vi "Calibratge.vi"() -> (1 "OK ?":bool)   [LabVIEW 2017]
uses:
  <vilib>/registry/registry.llb/Registry RtKey.ctl
  <vilib>/registry/registry.llb/Registry View.ctl
  <vilib>/registry/registry.llb/Write Registry Value Simple STR.vi
panel:
  in  "TermeInd 2":dbl caption="PendentCel2"
  out "TermesInd":dbl[](array[numeric]) caption="Pendents" format="%#_8g"
  in  "TermeInd 1":dbl caption="PendentCel1"
  in  "CALIBRAR":bool caption="ACTIVA CALIBRAR"
  in  "Idioma":string(combo)
  in  "ViuMotor":bool caption="Viu Motor Actiu"
  in  "MotorBipolar":bool caption="Motor Bipolar"
  in  "DeforActiva":bool
  in  "VelocitatMaxima":dbl caption="Velocitat Màxima"
  in  "ResoExten":i8(ring) caption="Resolució Extensometre" items=["0.1", "0.2", "0.5", "0.01", "0.02", "0.05", "0.001", "0.002", "0.005"]
  in  "Pendent_D":dbl caption="Extensometro" format="%#_8g"
  in  "Text Defor":string caption="Text defor"
  out "Unidades 2":i32[](array[numeric])
  in  "Unidades Célula 2":i32[](listbox) caption="Célula 2"
  out "Unidades 1":i32[](array[numeric])
  in  "Célula 2":u8(ring) items=["0.5 kg", "1 Kg", "2 Kg", "5 kg", "10 kg", "20 kg", "50 kg", "100 kg", "200 kg", "300 kg", "500 kg", "1000 kg", "2000 kg", "5000 kg", "10000 kg", "20000 kg", "30000 kg", "P-20 kg", "P-200 kg", "P-500 kg", "P-5000 kg", "P-20000 kg", "P-40 bar", "P-60 bar", "P- 20 bar", "No presente"]
  in  "Unidades Célula 1":i32[](listbox) caption="Célula 1"
  in  "SobrecargaC2":dbl
  in  "SobrecargaC1":dbl
  in  "C3-E2":u16(ring) items=["1", "2", "5", "10", "0.1", "0.01", "0.001", "0.0001", "0.5", "0.05", "0.005", "0.0005", "0.25", "0.025", "0.0025", "0.00025", "0.2", "0.02", "0.002", "0.0002"]
  in  "C2-E2":u16(ring) items=["1", "2", "5", "10", "0.1", "0.01", "0.001", "0.0001", "0.5", "0.05", "0.005", "0.0005", "0.25", "0.025", "0.0025", "0.00025", "0.2", "0.02", "0.002", "0.0002"]
  in  "C3-E1":u16(ring) items=["1", "2", "5", "10", "0.1", "0.01", "0.001", "0.0001", "0.5", "0.05", "0.005", "0.0005", "0.25", "0.025", "0.0025", "0.00025", "0.2", "0.02", "0.002", "0.0002"]
  in  "C2-E1":u16(ring) items=["1", "2", "5", "10", "0.1", "0.01", "0.001", "0.0001", "0.5", "0.05", "0.005", "0.0005", "0.25", "0.025", "0.0025", "0.00025", "0.2", "0.02", "0.002", "0.0002"]
  out "Célula 3":string
  in  "PendentCel3":dbl
  in  "PendentCel2":dbl
  in  "Número de Célules":dbl
  in  "TextTemps":string caption="Text temps"
  in  "Célula 1":i8(ring) items=["0.5 kg", "1 Kg", "2 Kg", "5 kg", "10 kg", "20 kg", "50 kg", "100 kg", "200 kg", "300 kg", "500 kg", "1000 kg", "2000 kg", "5000 kg", "10000 kg", "20000 kg", "30000 kg", "P-20 kg", "P-200 kg", "P-500 kg", "P-5000 kg", "P-20000 kg", "P-40 bar", "P-60 bar", "P-20 bar"]
  in  "PendentCel1":dbl
  in  "Password":string
  in  "error in (no error)":errorcluster
  out "Pendents":dbl[](array[numeric]) format="%#_8g"
  in  "Cancel":bool
  in  "OK Button":bool
  in  "Pendent_T":dbl caption="CaptadorD" format="%#_8g"
  # "Pendent"
  # "Sobrecarga"
  # "Ind."
  # "Pendent"
  # "Sobrecarga"
  # "Si vols modificar el password\nintrodueix-ne un de nou"
  # "Ind."
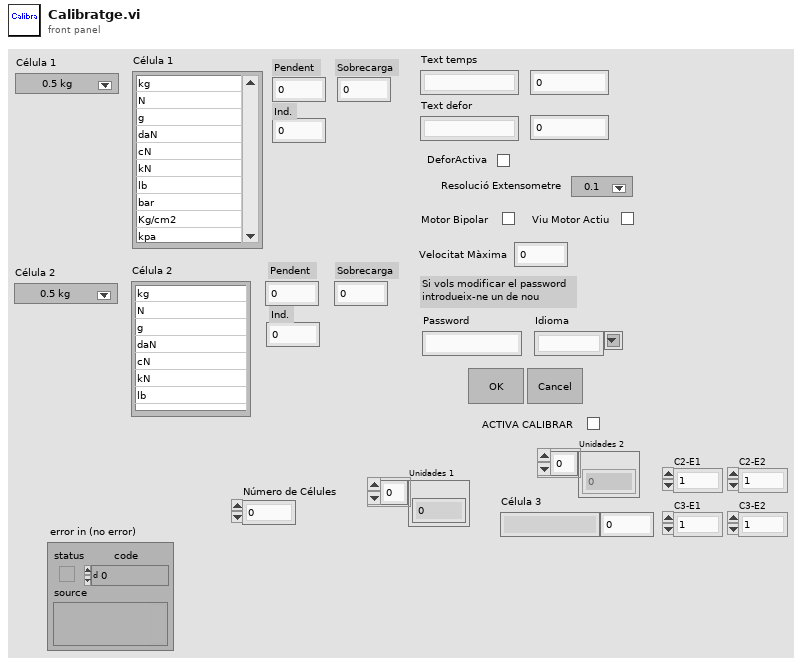
[diagram p1: front panel]
types:
  T1 = typedef "Registry RtKey.ctl" = enum32{"HKEY_CLASSES_ROOT", "HKEY_CURRENT_USER", "HKEY_LOCAL_MACHINE", "HKEY_USERS", "HKEY_PERFORMANCE_DATA", "HKEY_CURRENT_CONFIG", "HKEY_DYN_DATA"}
  T2 = typedef "Registry View.ctl" = u16
  T3 = typedef "Registry refnum.ctl" = refnum<k1>
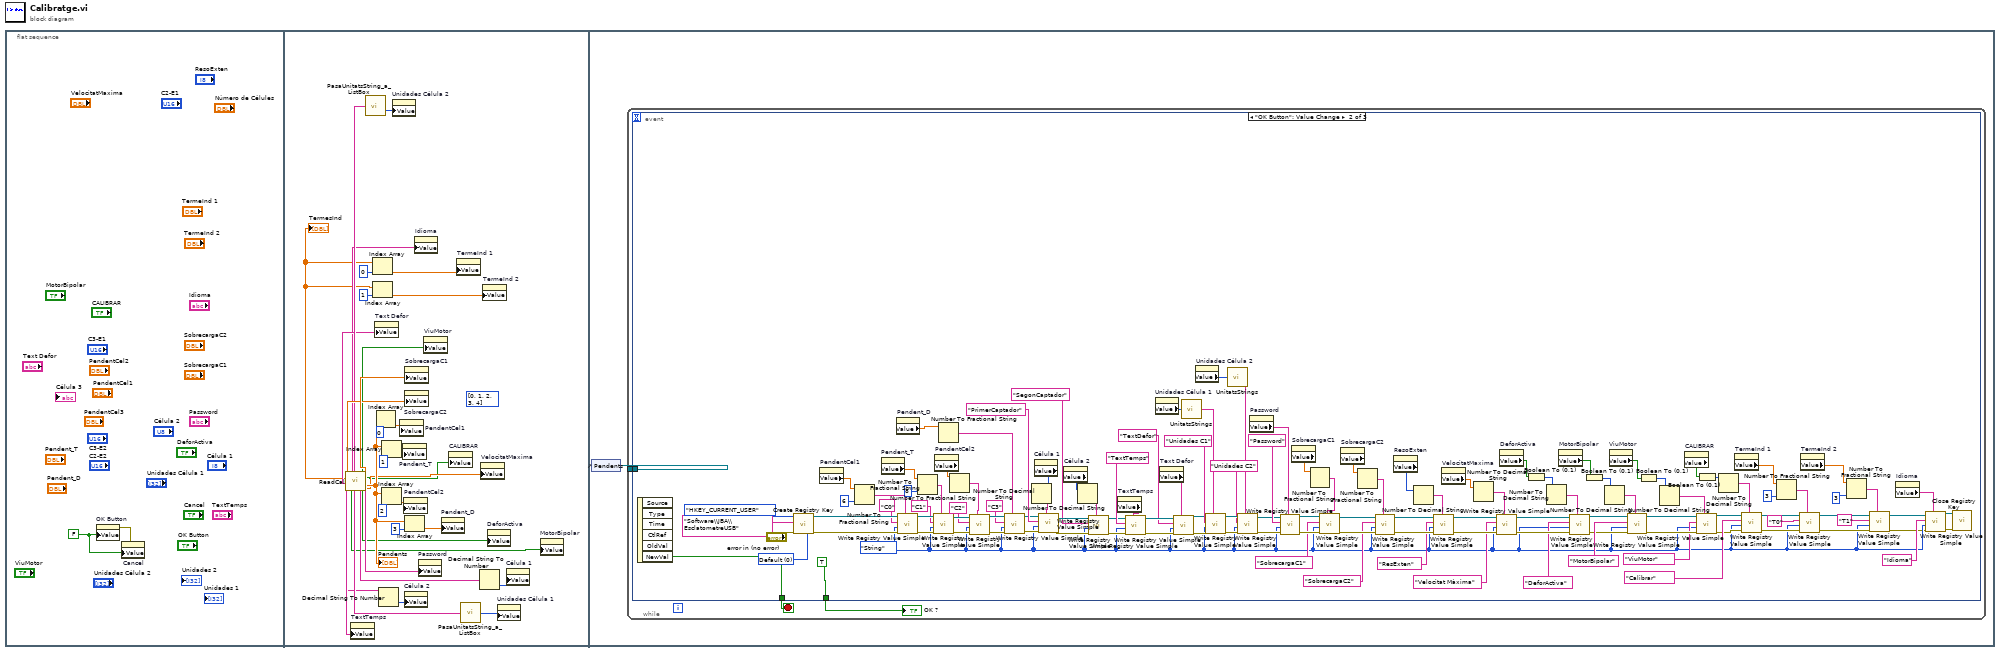
[diagram p0: block diagram]
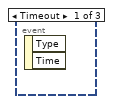
[diagram p2: hidden frame]
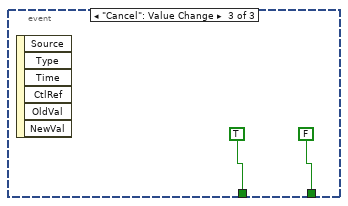
[diagram p3: hidden frame]
diagram:
  n1 = flat-sequence {
    frame #0 {
      w1 = FALSE ("OK Button")
      n2 = property on="OK Button" class="Bool (strict)"("Value"=w1) -> (error out=w2:errorcluster)  [unwired: 2 in, 1 out]
      n3 = property on="Cancel" class="Bool (strict)"(error in=w2, "Value"=w1) -> ()  [unwired: 1 in, 2 out]
    }
    frame #1 {
      (unwired) i32[] [0, 1, 2, 3, 4] ("Unidades 2")
      n4 = call "ReadCal.vi"() -> ("SobrecargaC2"=w27:dbl, "TermesInd"=w5:dbl[], "TextTemps"=w17:string, "TextDefor"=w26:string, "SegonCaptador"=w18:string, "Idioma"=w9:string, "MotorBipolar"=w11:bool, "UnitatsC2"=w25:string, "UnitatsC1"=w23:string, "PrimerCaptador"=w21:string, "ViuMotor"=w10:bool, "DeforActiva"=w12:bool, "Calibrar"=w8:bool, "SobrecargaC1"=w28:dbl, "Password"=w35:string, "Pendents"=w15:dbl[], "VelocitatMàxima"=w13:dbl)  [unwired: 2 in, 9 out]
      "Pendents" <- w15
      "TermesInd" <- w5
      n5 = property on="TextTemps" class="Str"("Value"=w26) -> ()  [unwired: 2 in, 2 out]
      n6 = call "PasaUnitatsString_a_ListBox.vi"("UnitatsC2"=w25) -> ("Value"=w24:i32[])
      n7 = Index Array(array=w5, index=0) -> (element=w4:dbl)
      n8 = Index Array(array=w5, index=1) -> (element=w3:dbl)
      n9 = property on="Text Defor" class="Str"("Value"=w17) -> ()  [unwired: 2 in, 2 out]
      n10 = Index Array(array=w15, index=0) -> (element=w33:dbl)
      n11 = Decimal String To Number(string=w18) -> (number=w19:i32)  [unwired: 2 in, 1 out]
      n12 = Index Array(array=w15, index=1) -> (element=w31:dbl)
      n13 = Index Array(array=w15, index=2) -> (element=w30:dbl)
      n14 = property on="Unidades Célula 2" class="LstBox (strict)"("Value"=w24) -> ()  [unwired: 2 in, 2 out]
      n15 = property on="PendentCel1" class="DigNum (strict)"("Value"=w33) -> ()  [unwired: 2 in, 2 out]
      n16 = property on="Pendent_T" class="DigNum (strict)"("Value"=w31) -> ()  [unwired: 2 in, 2 out]
      n17 = property on="PendentCel2" class="DigNum (strict)"("Value"=w30) -> ()  [unwired: 2 in, 2 out]
      n18 = property on="Célula 2" class="Ring (strict)"("Value"=w19) -> ()  [unwired: 2 in, 2 out]
      n19 = property on="SobrecargaC1" class="DigNum (strict)"("Value"=w28) -> ()  [unwired: 2 in, 2 out]
      n20 = property on="SobrecargaC2" class="DigNum (strict)"("Value"=w27) -> ()  [unwired: 2 in, 2 out]
      n21 = Index Array(array=w15, index=3) -> (element=w14:dbl)
      n22 = property on="Idioma" class="CmbBox"("Value"=w9) -> ()  [unwired: 2 in, 2 out]
      n23 = property on="Password" class="Str"("Value"=w35) -> ()  [unwired: 2 in, 2 out]
      n24 = property on="ViuMotor" class="Bool (strict)"("Value"=w10) -> ()  [unwired: 2 in, 2 out]
      n25 = property on="Pendent_D" class="DigNum (strict)"("Value"=w14) -> ()  [unwired: 2 in, 2 out]
      n26 = property on="CALIBRAR" class="Bool (strict)"("Value"=w8) -> ()  [unwired: 2 in, 2 out]
      n27 = property on="TermeInd 1" class="DigNum (strict)"("Value"=w4) -> ()  [unwired: 2 in, 2 out]
      n28 = call "PasaUnitatsString_a_ListBox.vi"("UnitatsC2"=w23) -> ("Value"=w22:i32[])
      n29 = Decimal String To Number(string=w21) -> (number=w20:i32)  [unwired: 2 in, 1 out]
      n30 = property on="VelocitatMaxima" class="DigNum (strict)"("Value"=w13) -> ()  [unwired: 2 in, 2 out]
      n31 = property on="TermeInd 2" class="DigNum (strict)"("Value"=w3) -> ()  [unwired: 2 in, 2 out]
      n32 = property on="DeforActiva" class="Bool (strict)"("Value"=w12) -> ()  [unwired: 2 in, 2 out]
      n33 = property on="Unidades Célula 1" class="LstBox (strict)"("Value"=w22) -> ()  [unwired: 2 in, 2 out]
      n34 = property on="Célula 1" class="Ring (strict)"("Value"=w20) -> ()  [unwired: 2 in, 2 out]
      n35 = property on="MotorBipolar" class="Bool (strict)"("Value"=w11) -> ()  [unwired: 2 in, 2 out]
    }
    frame #2 {
      n36 = control-ref of="Pendents"() -> (w36:refnum<vi>)
      n37 = while {
        tunnel: w36 -> [w38]
        stop <- w39 stop-if-true
        n38 = event shown="[1] \"OK Button\": Value Change" {
          selector: _ -> [_ _ _]
          dyn-events: _ -> [_ _ _]
          timeout: _ -> [_ _ _]
          tunnel: [_ w162 TRUE ("NewVal")] -> w39
          tunnel: [_ TRUE ("Ok?") FALSE ("Ok?")] -> w37
          tunnel: w38 -> [_ _ _]
          event Timeout {
            n39 = event-data() -> ()  [unwired: 1 in, 2 out]
          }
          event "OK Button": Value Change {
            w65 = T2 0 items=["Default"=0, "KEY_WOW64_64KEY"=8, "KEY_WOW64_32KEY"=9] ("registry view")
            w43 = enum16{"String", "Binary", "DWORD"}."String" ("simple data type")
            n40 = event-data() -> ("NewVal"=w162:bool)  [unwired: 1 in, 5 out]
            n41 = call <vilib>:"Create Registry Key.vi"("registry view"=w65, "error in (no error)"="error in (no error)", "subkey"="Software\\JBA\\EsclatometreUSB", "root key (HKEY_LOCAL_MACHINE)"=Registry_RtKey."HKEY_CURRENT_USER") -> ("error out"=w68:errorcluster, "refnum out"=w69:T3)  [unwired: 5 in, 1 out]
            n42 = property on="PendentCel1" class="DigNum (strict)"() -> ("Value"=w157:dbl)  [unwired: 2 in, 2 out]
            n43 = Number To Fractional String(number=w157, precision (6)=i16 6) -> (F-format string=w155:string)  [unwired: 2 in]
            n44 = property on="Pendent_T" class="DigNum (strict)"() -> ("Value"=w153:dbl)  [unwired: 2 in, 2 out]
            n45 = property on="Pendent_D" class="DigNum (strict)"() -> ("Value"=w113:dbl)  [unwired: 2 in, 2 out]
            n46 = call-poly <vilib>:"Write Registry Value Simple.vi"("String/Binary data"=w155, "error in (no error)"=w68, "simple data type"=w43, "value"="C0", "refnum"=w69) -> ("error out"=w160:errorcluster, "refnum out"=w159:T3)  [unwired: 3 in]
            n47 = Number To Fractional String(number=w153, precision (6)=i16 8) -> (F-format string=w154:string)  [unwired: 2 in]
            n48 = call-poly <vilib>:"Write Registry Value Simple.vi"("String/Binary data"=w154, "error in (no error)"=w160, "simple data type"=w43, "value"="C1", "refnum"=w159) -> ("error out"=w151:errorcluster, "refnum out"=w152:T3)  [unwired: 3 in]
            n49 = property on="PendentCel2" class="DigNum (strict)"() -> ("Value"=w149:dbl)  [unwired: 2 in, 2 out]
            n50 = Number To Fractional String(number=w113) -> (F-format string=w108:string)  [unwired: 3 in]
            n51 = Number To Fractional String(number=w149) -> (F-format string=w148:string)  [unwired: 3 in]
            n52 = call-poly <vilib>:"Write Registry Value Simple.vi"("String/Binary data"=w148, "error in (no error)"=w151, "simple data type"=w43, "value"="C2", "refnum"=w152) -> ("error out"=w112:errorcluster, "refnum out"=w111:T3)  [unwired: 3 in]
            n53 = call-poly <vilib>:"Write Registry Value Simple.vi"("String/Binary data"=w108, "error in (no error)"=w112, "simple data type"=w43, "value"="C3", "refnum"=w111) -> ("error out"=w109:errorcluster, "refnum out"=w110:T3)  [unwired: 3 in]
            n54 = property on="Célula 1" class="Ring (strict)"() -> ("Value"=w129:i8)  [unwired: 2 in, 2 out]
            n55 = Number To Decimal String(number=w129) -> (decimal integer string=w128:string)  [unwired: 1 in]
            n56 = call-poly <vilib>:"Write Registry Value Simple.vi"("String/Binary data"=w128, "error in (no error)"=w109, "simple data type"=w43, "value"="PrimerCaptador", "refnum"=w110) -> ("error out"=w145:errorcluster, "refnum out"=w146:T3)  [unwired: 3 in]
            n57 = property on="Célula 2" class="Ring (strict)"() -> ("Value"=w116:u8)  [unwired: 2 in, 2 out]
            n58 = Number To Decimal String(number=w116) -> (decimal integer string=w115:string)  [unwired: 1 in]
            n59 = call-poly <vilib>:"Write Registry Value Simple.vi"("String/Binary data"=w115, "error in (no error)"=w145, "simple data type"=w43, "value"="SegonCaptador", "refnum"=w146) -> ("error out"=w142:errorcluster, "refnum out"=w143:T3)  [unwired: 3 in]
            n60 = property on="TextTemps" class="Str"() -> ("Value"=w125:string)  [unwired: 2 in, 2 out]
            n61 = call-poly <vilib>:"Write Registry Value Simple.vi"("String/Binary data"=w125, "error in (no error)"=w142, "simple data type"=w43, "value"="TextTemps", "refnum"=w143) -> ("error out"=w104:errorcluster, "refnum out"=w105:T3)  [unwired: 3 in]
            n62 = property on="Unidades Célula 1" class="LstBox (strict)"() -> ("Value"=w127:i32[])  [unwired: 2 in, 2 out]
            n63 = property on="Text Defor" class="Str"() -> ("Value"=w101:string)  [unwired: 2 in, 2 out]
            n64 = call-poly <vilib>:"Write Registry Value Simple.vi"("String/Binary data"=w101, "error in (no error)"=w104, "simple data type"=w43, "value"="TextDefor", "refnum"=w105) -> ("error out"=w103:errorcluster, "refnum out"=w102:T3)  [unwired: 3 in]
            n65 = call "UnitatsStrings.vi"("UnidadesCelula"=w127) -> ("StringUnidades"=w124:string)
            n66 = property on="Unidades Célula 2" class="LstBox (strict)"() -> ("Value"=w123:i32[])  [unwired: 2 in, 2 out]
            n67 = call-poly <vilib>:"Write Registry Value Simple.vi"("String/Binary data"=w124, "error in (no error)"=w103, "simple data type"=w43, "value"="Unidades C1", "refnum"=w102) -> ("error out"=w121:errorcluster, "refnum out"=w122:T3)  [unwired: 3 in]
            n68 = call "UnitatsStrings.vi"("UnidadesCelula"=w123) -> ("StringUnidades"=w117:string)
            n69 = call-poly <vilib>:"Write Registry Value Simple.vi"("String/Binary data"=w117, "error in (no error)"=w121, "simple data type"=w43, "value"="Unidades C2", "refnum"=w122) -> ("error out"=w120:errorcluster, "refnum out"=w119:T3)  [unwired: 3 in]
            n70 = property on="Password" class="Str"() -> ("Value"=w141:string)  [unwired: 2 in, 2 out]
            n71 = call-poly <vilib>:"Write Registry Value Simple.vi"("String/Binary data"=w141, "error in (no error)"=w120, "simple data type"=w43, "value"="Password", "refnum"=w119) -> ("error out"=w138:errorcluster, "refnum out"=w137:T3)  [unwired: 3 in]
            n72 = property on="SobrecargaC1" class="DigNum (strict)"() -> ("Value"=w139:dbl)  [unwired: 2 in, 2 out]
            n73 = Number To Fractional String(number=w139) -> (F-format string=w133:string)  [unwired: 3 in]
            n74 = call-poly <vilib>:"Write Registry Value Simple.vi"("String/Binary data"=w133, "error in (no error)"=w138, "simple data type"=w43, "value"="SobrecargaC1", "refnum"=w137) -> ("error out"=w131:errorcluster, "refnum out"=w132:T3)  [unwired: 3 in]
            n75 = property on="SobrecargaC2" class="DigNum (strict)"() -> ("Value"=w135:dbl)  [unwired: 2 in, 2 out]
            n76 = Number To Fractional String(number=w135) -> (F-format string=w134:string)  [unwired: 3 in]
            n77 = call-poly <vilib>:"Write Registry Value Simple.vi"("String/Binary data"=w134, "error in (no error)"=w131, "simple data type"=w43, "value"="SobrecargaC2", "refnum"=w132) -> ("error out"=w97:errorcluster, "refnum out"=w98:T3)  [unwired: 3 in]
            n78 = property on="ResoExten" class="Ring (strict)"() -> ("Value"=w96:i8)  [unwired: 2 in, 2 out]
            n79 = Number To Decimal String(number=w96) -> (decimal integer string=w99:string)  [unwired: 1 in]
            n80 = call-poly <vilib>:"Write Registry Value Simple.vi"("String/Binary data"=w99, "error in (no error)"=w97, "simple data type"=w43, "value"="ResExten", "refnum"=w98) -> ("error out"=w93:errorcluster, "refnum out"=w94:T3)  [unwired: 3 in]
            n81 = property on="VelocitatMaxima" class="DigNum (strict)"() -> ("Value"=w90:dbl)  [unwired: 2 in, 2 out]
            n82 = Number To Decimal String(number=w90) -> (decimal integer string=w91:string)  [unwired: 1 in]
            n83 = call-poly <vilib>:"Write Registry Value Simple.vi"("String/Binary data"=w91, "error in (no error)"=w93, "simple data type"=w43, "value"="Velocitat Màxima", "refnum"=w94) -> ("error out"=w88:errorcluster, "refnum out"=w89:T3)  [unwired: 3 in]
            n84 = property on="DeforActiva" class="Bool (strict)"() -> ("Value"=w84:bool)  [unwired: 2 in, 2 out]
            n85 = Boolean To (0,1)(Boolean=w84) -> (0, 1=w87:i16)
            n86 = Number To Decimal String(number=w87) -> (decimal integer string=w86:string)  [unwired: 1 in]
            n87 = property on="MotorBipolar" class="Bool (strict)"() -> ("Value"=w80:bool)  [unwired: 2 in, 2 out]
            n88 = call-poly <vilib>:"Write Registry Value Simple.vi"("String/Binary data"=w86, "error in (no error)"=w88, "simple data type"=w43, "value"="DeforActiva", "refnum"=w89) -> ("error out"=w78:errorcluster, "refnum out"=w79:T3)  [unwired: 3 in]
            n89 = Boolean To (0,1)(Boolean=w80) -> (0, 1=w83:i16)
            n90 = Number To Decimal String(number=w83) -> (decimal integer string=w82:string)  [unwired: 1 in]
            n91 = property on="ViuMotor" class="Bool (strict)"() -> ("Value"=w74:bool)  [unwired: 2 in, 2 out]
            n92 = call-poly <vilib>:"Write Registry Value Simple.vi"("String/Binary data"=w82, "error in (no error)"=w78, "simple data type"=w43, "value"="MotorBipolar", "refnum"=w79) -> ("error out"=w76:errorcluster, "refnum out"=w77:T3)  [unwired: 3 in]
            n93 = Boolean To (0,1)(Boolean=w74) -> (0, 1=w75:i16)
            n94 = Number To Decimal String(number=w75) -> (decimal integer string=w73:string)  [unwired: 1 in]
            n95 = property on="CALIBRAR" class="Bool (strict)"() -> ("Value"=w59:bool)  [unwired: 2 in, 2 out]
            n96 = call-poly <vilib>:"Write Registry Value Simple.vi"("String/Binary data"=w73, "error in (no error)"=w76, "simple data type"=w43, "value"="ViuMotor", "refnum"=w77) -> ("error out"=w54:errorcluster, "refnum out"=w53:T3)  [unwired: 3 in]
            n97 = Boolean To (0,1)(Boolean=w59) -> (0, 1=w60:i16)
            n98 = Number To Decimal String(number=w60) -> (decimal integer string=w58:string)  [unwired: 1 in]
            n99 = property on="TermeInd 1" class="DigNum (strict)"() -> ("Value"=w49:dbl)  [unwired: 2 in, 2 out]
            n100 = call-poly <vilib>:"Write Registry Value Simple.vi"("String/Binary data"=w58, "error in (no error)"=w54, "simple data type"=w43, "value"="Calibrar", "refnum"=w53) -> ("error out"=w55:errorcluster, "refnum out"=w52:T3)  [unwired: 3 in]
            n101 = Number To Fractional String(number=w49, precision (6)=i16 3) -> (F-format string=w51:string)  [unwired: 2 in]
            n102 = call-poly <vilib>:"Write Registry Value Simple.vi"("String/Binary data"=w51, "error in (no error)"=w55, "simple data type"=w43, "value"="T0", "refnum"=w52) -> ("error out"=w44:errorcluster, "refnum out"=w45:T3)  [unwired: 3 in]
            n103 = property on="TermeInd 2" class="DigNum (strict)"() -> ("Value"=w42:dbl)  [unwired: 2 in, 2 out]
            n104 = Number To Fractional String(number=w42, precision (6)=i16 3) -> (F-format string=w47:string)  [unwired: 2 in]
            n105 = call-poly <vilib>:"Write Registry Value Simple.vi"("String/Binary data"=w47, "error in (no error)"=w44, "simple data type"=w43, "value"="T1", "refnum"=w45) -> ("error out"=w40:errorcluster, "refnum out"=w41:T3)  [unwired: 3 in]
            n106 = property on="Idioma" class="CmbBox"() -> ("Value"=w63:string)  [unwired: 2 in, 2 out]
            n107 = call-poly <vilib>:"Write Registry Value Simple.vi"("String/Binary data"=w63, "error in (no error)"=w40, "simple data type"=w43, "value"="Idioma", "refnum"=w41) -> ("error out"=w62:errorcluster, "refnum out"=w61:T3)  [unwired: 3 in]
            n108 = call <vilib>:"Close Registry Key.vi"("error in (no error)"=w62, "refnum"=w61) -> ()  [unwired: 5 in, 1 out]
          }
          event "Cancel": Value Change {
            n109 = event-data() -> ()  [unwired: 1 in, 6 out]
          }
        }
        "OK ?" <- w37
      }
    }
  }
